vi "Barra puntos.vi"(1 "#N":i32) -> (5 "String":string)   [LabVIEW 2019]
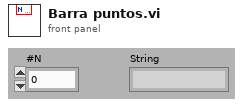
[diagram p1: front panel]
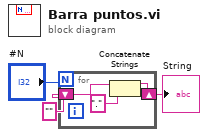
[diagram p0: block diagram]
diagram:
  n1 = for {
    N: "#N" -> [_]
    shift-right: [w4] -> w3
    shift-left: "" -> [w5]
    n2 = Concatenate Strings(w5, ".") -> (w4:string)
  }
  "String" <- w3
